vi "build unique object Insance name.vi"(11 "object instance prefix":string) -> (3 "object instance name":string)   [LabVIEW 2019, in "HLA Custom Device Engine.lvlib"]
uses:
  HLA Custom Device Engine.lvlib
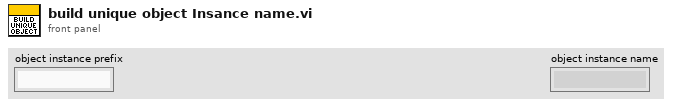
[diagram p1: front panel]
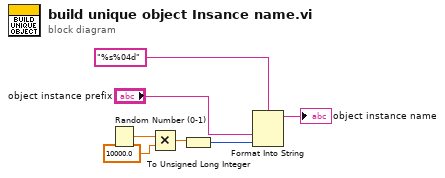
[diagram p0: block diagram]
diagram:
  n1 = Random Number (0-1)() -> (number: 0 to 1=w7:dbl)
  n2 = Multiply(x=w7, y=10000.0) -> (x*y=w6:dbl)
  n3 = To Unsigned Long Integer(number=w6) -> (unsigned 32bit integer=w5:u32)
  n4 = Format Into String(format string="%s%04d", "object instance prefix", w5) -> (resulting string=→"object instance name":string)  [unwired: 2 in, 1 out]
